vi "Mask Write Holding Register.vi"(4 "OR Mask":u16, 6 "AND Mask":u16, 7 "unit ID":u8, 8 "error in":errorcluster, 10 "address":u16, 11 "Modbus instance in":refnum<class "Modbus Master.lvclass">) -> (0 "error out":errorcluster, 3 "Modbus instance out":refnum<class "Modbus Master.lvclass">)   [LabVIEW 2013, in "Modbus Library - Advance.lvlib" / "Modbus Master.lvclass"]
doc: "Writes the masked value of a single register using an <b>AND mask</b> and an <b>OR mask</b> using the equation below:\nResult=(Current Value AND AndMask) OR (OrMask AND !AndMask)"
uses:
  Modbus Master.lvclass
  Modbus Master.lvclass/Modbus Master.ctl
  Modbus API.lvclass/Modbus API.ctl
  Transmission Data Unit/Transmission Data Unit.lvclass/Transmission Data Unit.ctl
  Transmission Data Unit/Transmission Data Unit.lvclass
  Master Function Definition/Master Function Definition.lvclass
  Modbus API.lvclass
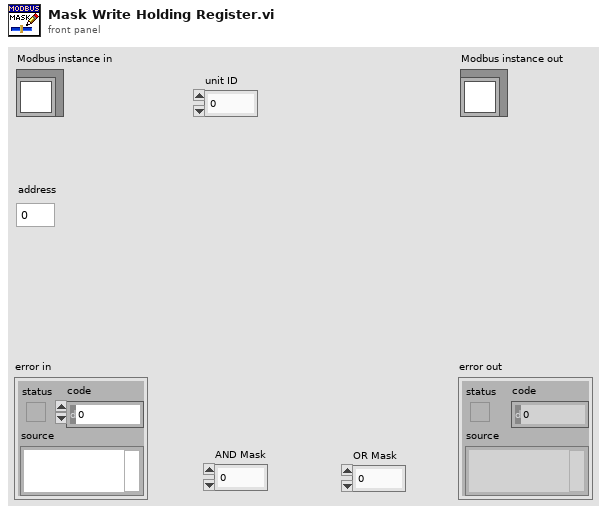
[diagram p1: front panel]
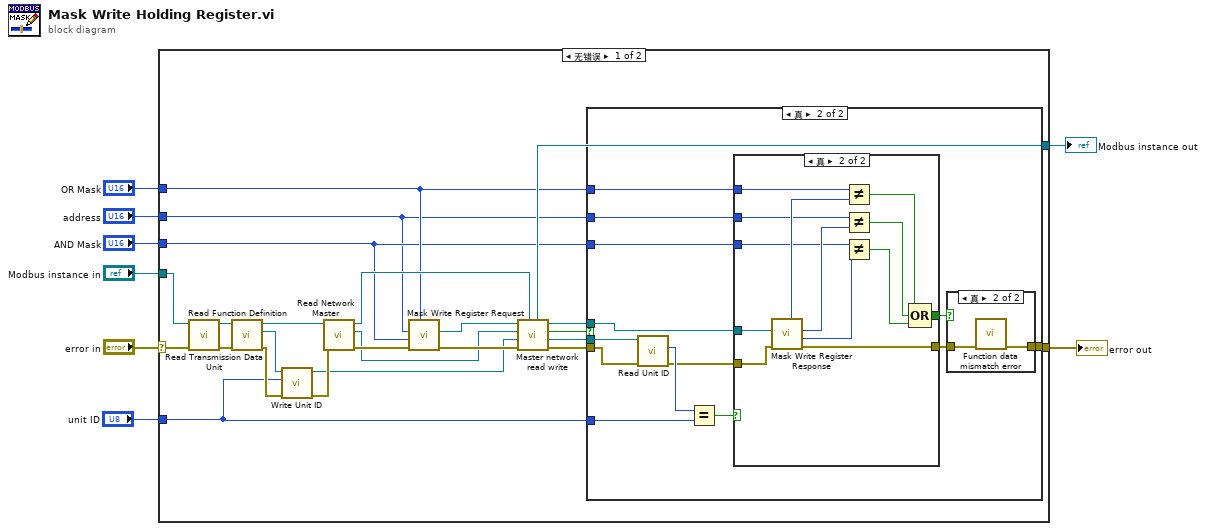
[diagram p0: block diagram]
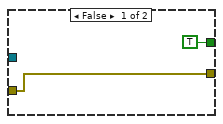
[diagram p3: hidden frame]
diagram:
  n1 = case shown="无错误" "error in" {
    selector: "error in" -> [w23 w65]
    tunnel: "Modbus instance in" -> [w21 w66]
    tunnel: [w27 w66] -> w7
    tunnel: [w31 w65] -> w6
    tunnel: "OR Mask" -> [w18 _]
    tunnel: "address" -> [w16 _]
    tunnel: "AND Mask" -> [w17 _]
    tunnel: "unit ID" -> [w10 _]
    frame No Error {
      n2 = call "Read Function Definition.vi"("error in"=w23, "Modbus master in"=w21) -> ("error out"=w25:errorcluster, "Modbus master out"=w24:refnum<class "Modbus Master.lvclass">)  [unwired: 7 in, 1 out]
      n3 = call "Read Transmission Data Unit.vi"("error in"=w25, "Modbus instance in"=w24) -> ("error out"=w13:errorcluster, "transmission data unit"=w14:refnum<class "Transmission Data Unit.lvclass">, "Modbus instance out"=w26:refnum<class "Modbus Master.lvclass">)  [unwired: 7 in]
      n4 = call "Write Unit ID.vi"("error in"=w13, "unit ID"=w10, "transmission data unit in"=w14) -> ("error out"=w12:errorcluster, "transmission data unit out"=w11:refnum<class "Transmission Data Unit.lvclass">)  [unwired: 7 in]
      n5 = call "Read Network Master.vi"("error in"=w12, "Modbus master in"=w26) -> ("error out"=w22:errorcluster, "network master"=w19:refnum<class "Network Master.lvclass">, "Modbus master out"=w20:refnum<class "Modbus Master.lvclass">)  [unwired: 7 in]
      n6 = call "Mask Write Register Request.vi"("OR mask"=w18, "error in"=w22, "AND mask"=w17, "Starting Address"=w16) -> ("error out"=w32:errorcluster, "modbus data unit out"=w29:refnum<class "Modbus Data Unit.lvclass">)  [unwired: 6 in]
      n7 = call "Master network read write.vi"("Modbus master in"=w20, "error in"=w32, "transmission data unit in"=w11, "network master in"=w19, "Modbus data unit in"=w29) -> ("error out"=w30:errorcluster, "transmission data unit out"=w9:refnum<class "Transmission Data Unit.lvclass">, "PDU Valid?"=w15:bool, "Modbus data unit out"=w28:refnum<class "Modbus Data Unit.lvclass">, "Modbus master out"=w27:refnum<class "Modbus Master.lvclass">)  [unwired: 2 in]
      n8 = case shown="真" w15 {
        tunnel: [w33 w45] -> w31
        tunnel: w30 -> [w33 w38]
        tunnel: w28 -> [_ w44]
        tunnel: w18 -> [_ w42]
        tunnel: w17 -> [_ w41]
        tunnel: w16 -> [_ w40]
        tunnel: w10 -> [_ w36]
        tunnel: w9 -> [_ w39]
        frame False {
        }
        frame True {
          n9 = call "Read Unit ID.vi"("error in"=w38, "transmission data unit in"=w39) -> ("error out"=w34:errorcluster, "unit ID"=w37:u8)  [unwired: 7 in, 1 out]
          n10 = Equal?(x=w37, y=w36) -> (x = y?=w35:bool)
          n11 = case shown="真" w35 {
            tunnel: [TRUE w60] -> w46
            tunnel: w44 -> [_ w57]
            tunnel: [w48 w56] -> w43
            tunnel: w42 -> [_ w52]
            tunnel: w41 -> [_ w51]
            tunnel: w40 -> [_ w50]
            tunnel: w34 -> [w48 w49]
            frame False {
            }
            frame True {
              n12 = call "Mask Write Register Response.vi"("error in"=w49, "modbus data unit in"=w57) -> ("error out"=w56:errorcluster, "AND mask"=w58:u16, "Address"=w59:u16, "OR mask"=w53:u16)  [unwired: 6 in]
              n13 = Not Equal?(x=w52, y=w53) -> (x != y?=w54:bool)
              n14 = Not Equal?(x=w50, y=w59) -> (x != y?=w55:bool)
              n15 = Not Equal?(x=w51, y=w58) -> (x != y?=w61:bool)
              n16 = Compound Arithmetic op=OR(w54, w55, w61) -> (w60:bool)
            }
          }
          n17 = case shown="真" w46 {
            tunnel: [w62 w64] -> w45
            tunnel: w43 -> [w62 w63]
            frame False {
            }
            frame True {
              n18 = call "Function data mismatch error.vi"("error in (no error)"=w63) -> ("error out"=w64:errorcluster)  [unwired: 10 in]
            }
          }
        }
      }
    }
    frame Error {
    }
  }
  "error out" <- w6
  "Modbus instance out" <- w7
